vi "outputSignal.vi"(8 "error in":errorcluster caption="errorIn", 11 "xmlRef":refnum<k20>) -> (0 "error out":errorcluster caption="errorOut", 3 "outputSignal":T1[](array[typedef]))   [LabVIEW 2017]
uses:
  models/TCN_outputSignal.ctl
  models/TCN_attachedInformation.ctl
  models/TCN_triggerConditions.ctl
  models/TCN_orSignals.ctl
  models/TCN_andSignals.ctl
  models/TCN_pulseClass.ctl
  <vilib>/xml/Close Reference(Node).vi
  <vilib>/xml/Close Reference(NdList).vi
  <resource>/objmgr/DOMUserDefRef.rc
  <vilib>/xml/NI_XML.lvlib
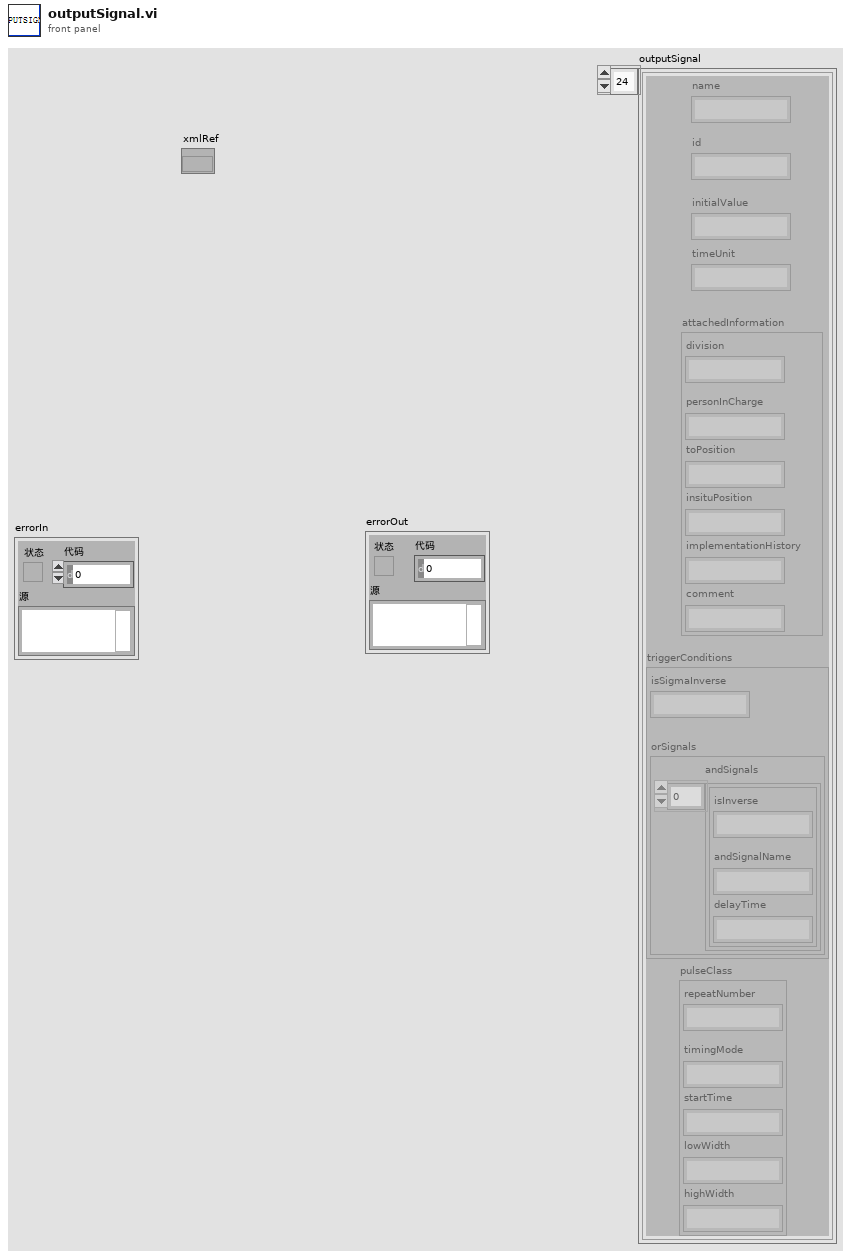
[diagram p1: front panel]
types:
  T1 = typedef "TCN_outputSignal.ctl" = cluster{"name":string, "id":string, "initialValue":string, "timeUnit":string, "attachedInformation":T2, "triggerConditions":T3, "pulseClass":T6}
  T2 = typedef "TCN_attachedInformation.ctl" = cluster{"division":string, "personInCharge":string, "toPosition":string, "insituPosition":string, "implementationHistory":string, "comment":string}
  T3 = typedef "TCN_triggerConditions.ctl" = cluster{"isSigmaInverse":string, "orSignals":T4}
  T4 = typedef "TCN_orSignals.ctl" = cluster{"andSignals":T5[]}
  T5 = typedef "TCN_andSignals.ctl" = cluster{"isInverse":string, "andSignalName":string, "delayTime":string}
  T6 = typedef "TCN_pulseClass.ctl" = cluster{"repeatNumber":string, "timingMode":string, "startTime":string, "lowWidth":string, "highWidth":string}
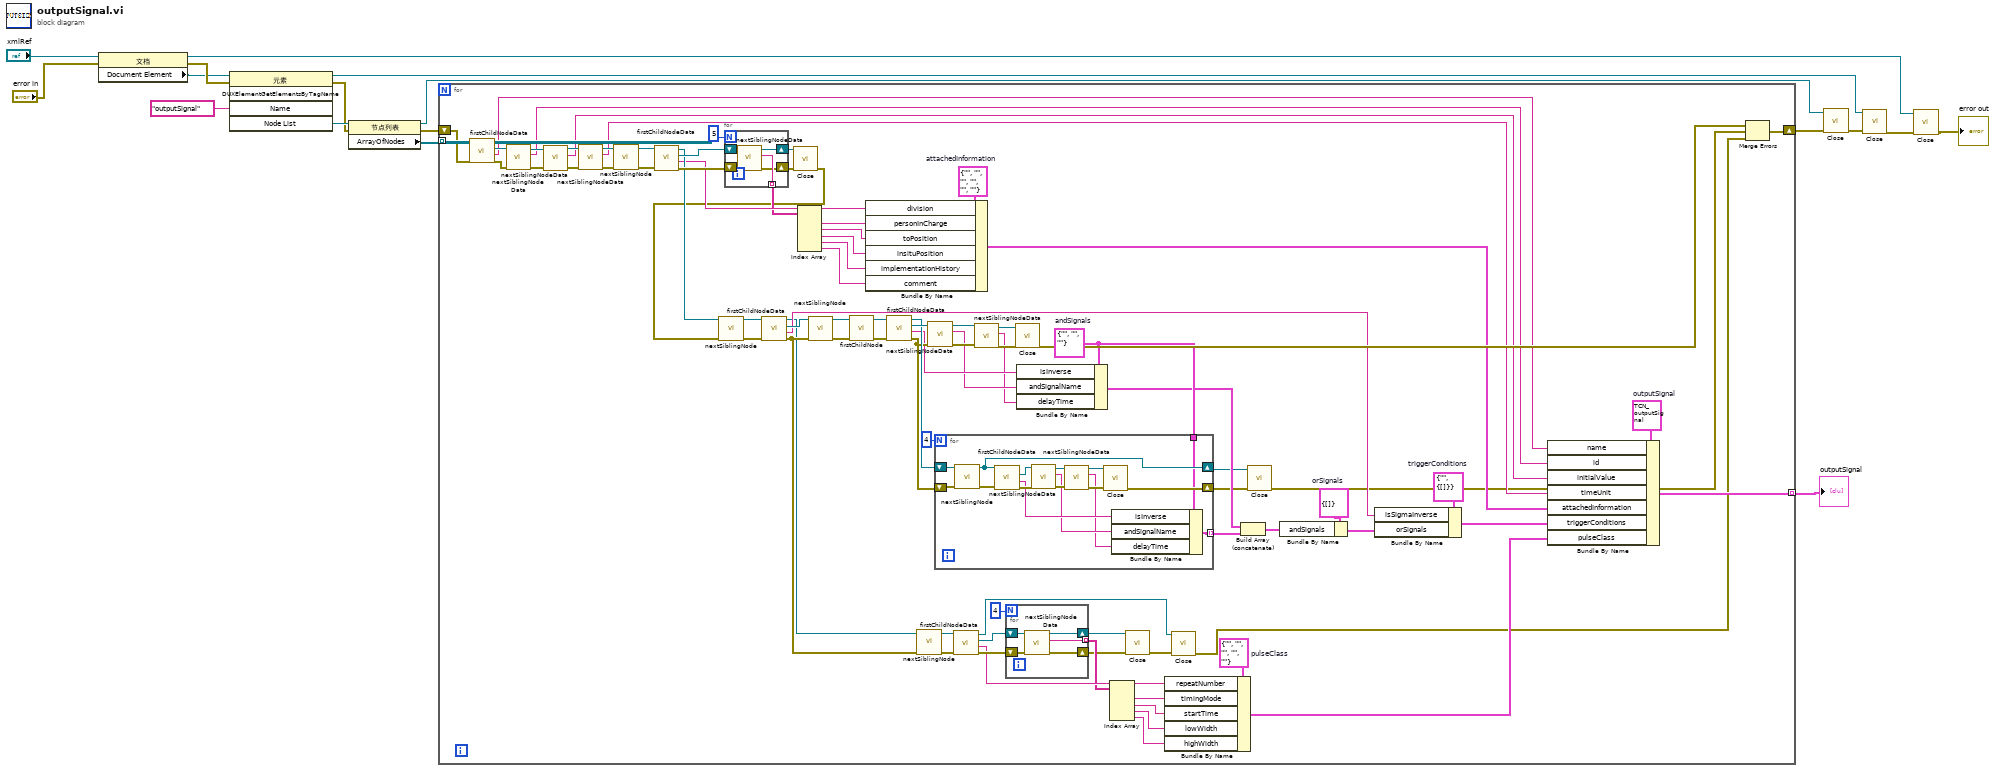
[diagram p0: block diagram]
diagram:
  n1 = property class="文档"(reference="xmlRef", error in="error in") -> (reference out=w1:refnum<k20>, error out=w16:errorcluster, "Document Element"=w15:refnum<k20>)
  n2 = invoke class="元素" method="DUXElementGetElementsByTagName"(reference=w15, error in=w16, "Name"="outputSignal" ("Node Name")) -> (reference out=w9:refnum<k20>, error out=w7:errorcluster, "Node List"=w8:refnum<k20>)  [unwired: 2 in, 2 out]
  n3 = property class="节点列表"(reference=w8, error in=w7) -> (reference out=w12:refnum<k20>, error out=w13:errorcluster, "ArrayOfNodes"=w14:refnum<k20>[])
  n4 = for {
    tunnel: w14 -> [w103] mode=indexing
    shift-right: [w67] -> w10
    shift-left: w13 -> [w72]
    tunnel: [w31] -> w5 mode=indexing
    w39 = T1 {"name"="", "id"="", "initialValue"="", "timeUnit"="", "attachedInformation"={"division"="", "personInCharge"="", "toPosition"="", "insituPosition"="", "implementationHistory"="", "comment"=""}, "triggerConditions"={"isSigmaInverse"="", "orSignals"={"andSignals"=[]}}, "pulseClass"={"repeatNumber"="", "timingMode"="", "startTime"="", "lowWidth"="", "highWidth"=""}}  # outputSignal
    w42 = T3 {"isSigmaInverse"="", "orSignals"={"andSignals"=[]}}  # triggerConditions
    w44 = T4 {"andSignals"=[]}  # orSignals
    w51 = T6 {"repeatNumber"="", "timingMode"="", "startTime"="", "lowWidth"="", "highWidth"=""}  # pulseClass
    w59 = T2 {"division"="", "personInCharge"="", "toPosition"="", "insituPosition"="", "implementationHistory"="", "comment"=""}  # attachedInformation
    w62 = T5 {"isInverse"="", "andSignalName"="", "delayTime"=""}  # andSignals
    n5 = call "firstChildNodeData.vi"("error in (no error)"=w72, "parentNode"=w103) -> ("error out"=w71:errorcluster, "data"=w38:string, "childNode"=w102:refnum<k20>)  [unwired: 6 in, 1 out]
    n6 = call "nextSiblingNodeData.vi"("error in (no error)"=w71, "siblingNode"=w102) -> ("error out"=w100:errorcluster, "data"=w37:string, "childNode"=w101:refnum<k20>)  [unwired: 7 in]
    n7 = call "nextSiblingNodeData.vi"("error in (no error)"=w100, "siblingNode"=w101) -> ("error out"=w98:errorcluster, "data"=w36:string, "childNode"=w99:refnum<k20>)  [unwired: 7 in]
    n8 = call "nextSiblingNodeData.vi"("error in (no error)"=w98, "siblingNode"=w99) -> ("error out"=w97:errorcluster, "data"=w35:string, "childNode"=w96:refnum<k20>)  [unwired: 7 in]
    n9 = call "nextSiblingNode.vi"("error in (no error)"=w97, "siblingNode"=w96) -> ("error out"=w85:errorcluster, "siblingNode"=w95:refnum<k20>)  [unwired: 7 in, 1 out]
    n10 = call "firstChildNodeData.vi"("error in (no error)"=w85, "parentNode"=w95) -> ("error out"=w84:errorcluster, "data"=w58:string, "childNode"=w90:refnum<k20>, "parentNode"=w82:refnum<k20>)  [unwired: 6 in]
    n11 = for {
      N: 5 -> [_]
      shift-right: [w127] -> w29
      shift-left: w90 -> [w129]
      tunnel: [w126] -> w57 mode=indexing
      shift-right: [w125] -> w30
      shift-left: w84 -> [w128]
      n12 = call "nextSiblingNodeData.vi"("error in (no error)"=w128, "siblingNode"=w129) -> ("error out"=w125:errorcluster, "data"=w126:string, "childNode"=w127:refnum<k20>)  [unwired: 7 in]
    }
    n13 = call-poly <vilib>:"Close.vi"("error in (no error)"=w30, "node"=w29) -> ("error out"=w28:errorcluster)  [unwired: 7 in]
    n14 = call "nextSiblingNode.vi"("error in (no error)"=w28, "siblingNode"=w82) -> ("error out"=w94:errorcluster, "siblingNode"=w88:refnum<k20>)  [unwired: 7 in, 1 out]
    n15 = call "firstChildNodeData.vi"("error in (no error)"=w94, "parentNode"=w88) -> ("error out"=w69:errorcluster, "data"=w41:string, "childNode"=w76:refnum<k20>, "parentNode"=w25:refnum<k20>)  [unwired: 6 in]
    n16 = Index Array(array=w57) -> (element #1=w56:string, element #2=w55:string, element #3=w54:string, element #4=w53:string, element #5=w52:string)  [unwired: 5 in]
    n17 = call "nextSiblingNode.vi"("error in (no error)"=w69, "siblingNode"=w76) -> ("error out"=w81:errorcluster, "siblingNode"=w93:refnum<k20>)  [unwired: 7 in, 1 out]
    n18 = call "firstChildNode.vi"("error in (no error)"=w81, "parentNode"=w93) -> ("error out"=w77:errorcluster, "childNode"=w79:refnum<k20>)  [unwired: 7 in, 1 out]
    n19 = Bundle By Name(cluster=w59, "division"=w58, "personInCharge"=w56, "toPosition"=w55, "insituPosition"=w54, "implementationHistory"=w53, "comment"=w52) -> (w34:T2)
    n20 = call "firstChildNodeData.vi"("error in (no error)"=w77, "parentNode"=w79) -> ("error out"=w70:errorcluster, "data"=w65:string, "childNode"=w89:refnum<k20>, "parentNode"=w78:refnum<k20>)  [unwired: 6 in]
    n21 = call "nextSiblingNode.vi"("error in (no error)"=w69, "siblingNode"=w25) -> ("error out"=w87:errorcluster, "siblingNode"=w86:refnum<k20>)  [unwired: 7 in, 1 out]
    n22 = call "nextSiblingNodeData.vi"("error in (no error)"=w70, "siblingNode"=w89) -> ("error out"=w91:errorcluster, "data"=w64:string, "childNode"=w92:refnum<k20>)  [unwired: 7 in]
    n23 = for {
      N: 4 -> [_]
      shift-right: [w118] -> w18
      shift-left: w78 -> [w124]
      shift-right: [w114] -> w19
      shift-left: w70 -> [w115]
      tunnel: w62 -> [w113]
      tunnel: [w109] -> w61 mode=indexing
      n24 = call "nextSiblingNode.vi"("error in (no error)"=w115, "siblingNode"=w124) -> ("error out"=w119:errorcluster, "siblingNode"=w118:refnum<k20>)  [unwired: 7 in, 1 out]
      n25 = call "firstChildNodeData.vi"("error in (no error)"=w119, "parentNode"=w118) -> ("error out"=w122:errorcluster, "data"=w112:string, "childNode"=w123:refnum<k20>)  [unwired: 6 in, 1 out]
      n26 = call "nextSiblingNodeData.vi"("error in (no error)"=w122, "siblingNode"=w123) -> ("error out"=w121:errorcluster, "data"=w111:string, "childNode"=w120:refnum<k20>)  [unwired: 7 in]
      n27 = call "nextSiblingNodeData.vi"("error in (no error)"=w121, "siblingNode"=w120) -> ("error out"=w117:errorcluster, "data"=w110:string, "childNode"=w116:refnum<k20>)  [unwired: 7 in]
      n28 = call-poly <vilib>:"Close.vi"("error in (no error)"=w117, "node"=w116) -> ("error out"=w114:errorcluster)  [unwired: 7 in]
      n29 = Bundle By Name(cluster=w113, "isInverse"=w112, "andSignalName"=w111, "delayTime"=w110) -> (w109:T5)
    }
    n30 = call "firstChildNodeData.vi"("error in (no error)"=w87, "parentNode"=w86) -> ("error out"=w68:errorcluster, "data"=w50:string, "childNode"=w24:refnum<k20>, "parentNode"=w21:refnum<k20>)  [unwired: 6 in]
    n31 = call "nextSiblingNodeData.vi"("error in (no error)"=w91, "siblingNode"=w92) -> ("error out"=w74:errorcluster, "data"=w63:string, "childNode"=w73:refnum<k20>)  [unwired: 7 in]
    n32 = for {
      N: 4 -> [_]
      shift-right: [w107] -> w27
      shift-left: w24 -> [w108]
      tunnel: [w106] -> w49 mode=indexing
      shift-right: [w105] -> w26
      shift-left: w68 -> [w104]
      n33 = call "nextSiblingNodeData.vi"("error in (no error)"=w104, "siblingNode"=w108) -> ("error out"=w105:errorcluster, "data"=w106:string, "childNode"=w107:refnum<k20>)  [unwired: 7 in]
    }
    n34 = call-poly <vilib>:"Close.vi"("error in (no error)"=w74, "node"=w73) -> ("error out"=w66:errorcluster)  [unwired: 7 in]
    n35 = Bundle By Name(cluster=w62, "isInverse"=w65, "andSignalName"=w64, "delayTime"=w63) -> (w60:T5)
    n36 = Index Array(array=w49) -> (element #1=w48:string, element #2=w47:string, element #3=w46:string, element #4=w45:string)  [unwired: 4 in]
    n37 = call-poly <vilib>:"Close.vi"("error in (no error)"=w26, "node"=w27) -> ("error out"=w23:errorcluster)  [unwired: 7 in]
    n38 = Bundle By Name(cluster=w51, "repeatNumber"=w50, "timingMode"=w48, "startTime"=w47, "lowWidth"=w46, "highWidth"=w45) -> (w32:T6)
    n39 = call-poly <vilib>:"Close.vi"("error in (no error)"=w23, "node"=w21) -> ("error out"=w22:errorcluster)  [unwired: 7 in]
    n40 = Build Array (concatenate)(w60, w61) -> (w43:T5[])
    n41 = call-poly <vilib>:"Close.vi"("error in (no error)"=w19, "node"=w18) -> ("error out"=w20:errorcluster)  [unwired: 7 in]
    n42 = Bundle By Name(cluster=w44, "andSignals"=w43) -> (w40:T4)
    n43 = Bundle By Name(cluster=w42, "isSigmaInverse"=w41, "orSignals"=w40) -> (w33:T3)
    n44 = Bundle By Name(cluster=w39, "name"=w38, "id"=w37, "initialValue"=w36, "timeUnit"=w35, "attachedInformation"=w34, "triggerConditions"=w33, "pulseClass"=w32) -> (w31:T1)
    n45 = Merge Errors(w66, w20, w22) -> (w67:errorcluster)
  }
  "outputSignal" <- w5
  n46 = call-poly <vilib>:"Close.vi"("error in (no error)"=w10, "node list"=w12) -> ("error out"=w11:errorcluster)  [unwired: 7 out]
  n47 = call-poly <vilib>:"Close.vi"("error in (no error)"=w11, "node"=w9) -> ("error out"=w3:errorcluster)  [unwired: 7 out]
  n48 = call-poly <vilib>:"Close.vi"("error in (no error)"=w3, "node"=w1) -> ("error out"=→"error out":errorcluster)  [unwired: 7 out]
